vi "Overwrite-all-gui-params.vi"(8 "error in (no error)":errorcluster, 10 "Mapping params.":T1={"Enable mapping"=FALSE, "Automatic timing"=FALSE, "Scan pattern file"=path "C:/CameraVision/Scan patterns/Template.sp", "Start off-set"=0.0, "Default map characteristic"=enum."Average intensity [0-255]", "Default mark speed"=1000, "Jump speed"=10000} {"Jump speed" min=1; "Default mark speed" min=1; "Start off-set" step=0.0001}, 11 "Mapping params. ref. in":refnum<data-value>) -> (0 "error out":errorcluster, 3 "Mapping params. ref.":refnum<data-value>)   [LabVIEW 2013, in "CameraVision.lvlib" / "CV-Mapping.lvclass"]
uses:
  CV-Mapping.lvclass
  Mapping-parameters-gui.ctl
  Mapping-characteristic.ctl
  CV-Mapping.lvclass/CV-Mapping.ctl
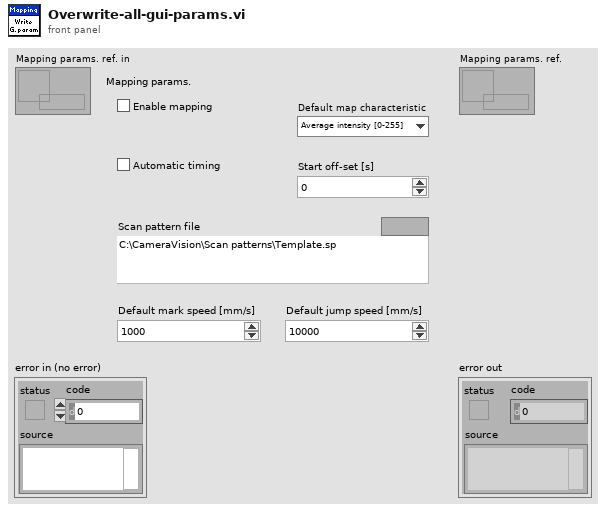
[diagram p1: front panel]
types:
  T1 = typedef "CameraVision.lvlib/CV-Mapping.lvclass/Mapping-parameters-gui.ctl" = cluster{"Enable mapping":bool, "Automatic timing":bool, "Scan pattern file":path, "Start off-set":dbl, "Default map characteristic":T2, "Default mark speed":i32, "Jump speed":i32}
  T2 = typedef "CameraVision.lvlib/CV-Mapping.lvclass/Mapping-characteristic.ctl" = enum16{"Average intensity [0-255]", "Peak intensity [0-255]", "Melt-pool size [mm²]", "Melt-pool aspect ratio []", "Melt-pool fragments []", "Average temperature [°C]", "Max. temperature [°C]", "Min. temperature [°C]", "Std. dev. temperature [°C]"}
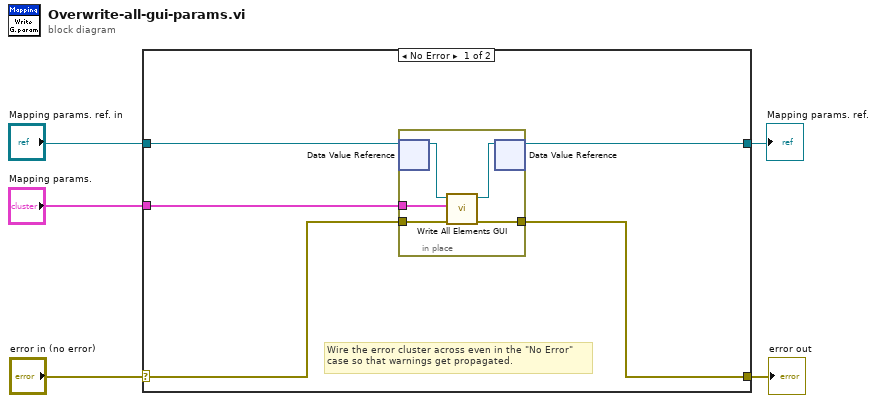
[diagram p0: block diagram]
diagram:
  n1 = case shown="No Error" "error in (no error)" {
    selector: "error in (no error)" -> [w8 w17]
    tunnel: [w10 w17] -> w4
    tunnel: "Mapping params. ref. in" -> [w7 w16]
    tunnel: "Mapping params." -> [w9 _]
    tunnel: [w6 w16] -> w1
    frame No Error {
      # "Wire the error cluster across even in the \"No Error\"\ncase so that warnings get propagated."
      n2 = in-place {
        in-place-border: [w15] -> w10
        in-place-border: w9 -> [w14]
        in-place-border: w8 -> [w13]
        n3 = in-place-dvr #1(w7) -> (w11:refnum<class "CV-Mapping.lvclass">)  [unwired: 1 out]
        n4 = call "Write All Elements GUI.vi"("error in (no error)"=w13, "Mapping params."=w14, "Mapping params in"=w11) -> ("error out"=w15:errorcluster, "Mapping params out"=w12:refnum<class "CV-Mapping.lvclass">)  [unwired: 7 in]
        n5 = in-place-dvr #1(w12) -> (w6:refnum<data-value>)  [unwired: 1 out]
      }
    }
    frame Error {
    }
  }
  "error out" <- w4
  "Mapping params. ref." <- w1
